vi "Get Base Protocol.vi"(8 "error in (no error)":errorcluster, 11 "Network Device in":refnum<class "Network Device.lvclass">=refnum) -> (0 "error out":errorcluster, 2 "Protocol out":T1, 3 "Network Device out":refnum<class "Network Device.lvclass">)   [LabVIEW 2019, in "Network Device.lvclass"]
uses:
  Network Device.lvclass
  Protocol Parent/Types/Base Protocol Type.ctl
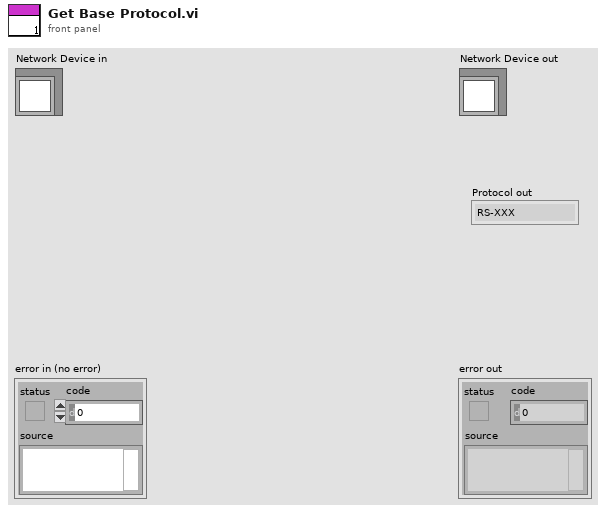
[diagram p1: front panel]
types:
  T1 = typedef "Protocol Classes.lvlib/Protocol Parent.lvclass/Base Protocol Type.ctl" = enum16{"RS-XXX", "VISA", "TCPIP", "UDP"}
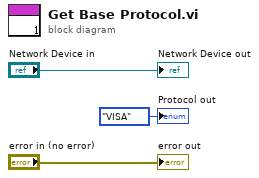
[diagram p0: block diagram]
diagram:
  "error out" <- "error in (no error)"
  "Network Device out" <- "Network Device in"
  "Protocol out" <- Base_Protocol_Type."VISA" ("Protocol out")
